vi "GetIntegrationTime.vi"(6 "Delay between send and receive [ms]":i32=100, 8 "error in (no error)":errorcluster, 11 "SCD in":refnum<class "SCD.lvclass">) -> (0 "error out":errorcluster, 2 "integration_time":i32, 3 "SCD out":refnum<class "SCD.lvclass">)   [LabVIEW 2023, in "horiba.lvlib" / "SCD.lvclass"]
doc: "Gets the integration time that was previously set. If no integration time has been explicitly set, the default value is returned.\nThe integration time is returned in seconds."
uses:
  SCD.lvclass
  b6349250-cb33-415b-847a-a7f5d99734f6.vi
  a3575502-22b1-481e-8bb0-96f3cfd6d110.vi
  <vilib>/JDP Science/JSONtext/Variant to JSON Text.vi
  <vilib>/JDP Science/JSONtext/Set Item.vi
  <vilib>/JDP Science/JSONtext/JSON text to Variant.vi
  <vilib>/JDP Science/JSONtext/LVClass Serializer/JSONtext LVClass Serializer.lvclass
  SCD.lvclass/SCD.ctl
  GenericDevice/GenericDevice.lvclass
panel:
  # "Connector Pane"
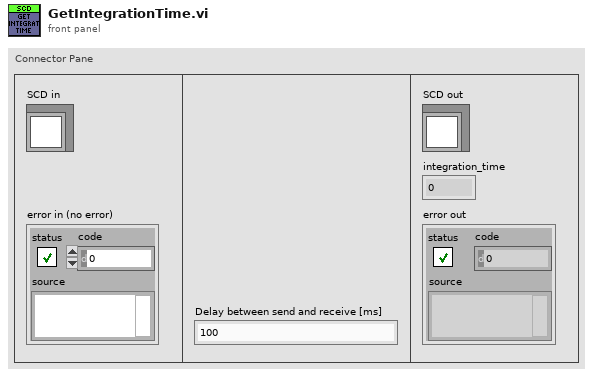
[diagram p1: front panel]
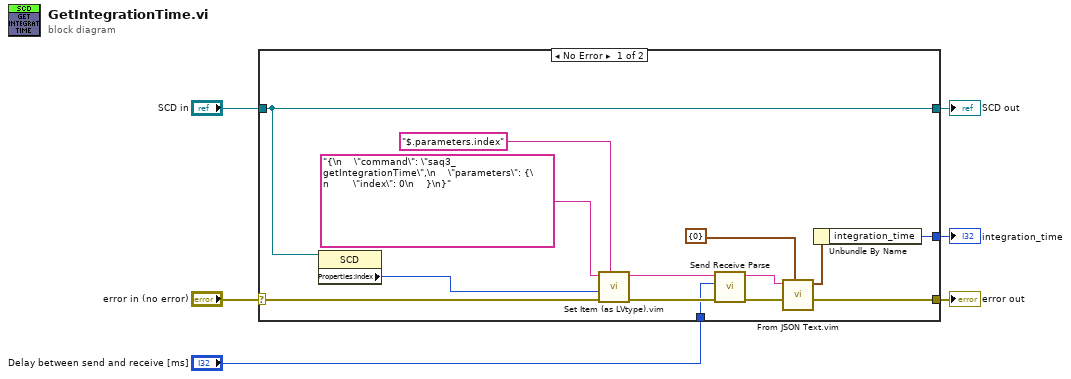
[diagram p0: block diagram]
diagram:
  n1 = case shown="No Error" "error in (no error)" {
    selector: "error in (no error)" -> [w16 w22]
    tunnel: [w15 w22] -> w2
    tunnel: [w18 w21] -> w4
    tunnel: "SCD in" -> [w18 w21]
    tunnel: [w10 _] -> w1
    tunnel: "Delay between send and receive [ms]" -> [w9 _]
    frame No Error {
      n2 = property class="SCD"(reference=w18) -> ("Properties:Index"=w17:i32)  [unwired: 1 in, 2 out]
      n3 = call "Set Item (as LVtype).vim"("$Path or Item Name"="$.parameters.index", "error in (no error)"=w16, "Anything"=w17, "JSON"="{\n    \"command\": \"saq3_getIntegrationTime\",\n    \"parameters\": {\n        \"index\": 0\n    }\n}") -> ("error out"=w13:errorcluster, "<JSON>"=w8:string)  [unwired: 4 in, 1 out]
      n4 = call "Send Receive Parse.vi"("error in"=w13, "Delay between send and receive [ms]"=w9, "<JSON>"=w8) -> ("error out"=w12:errorcluster, "results-JSON string"=w14:string)  [unwired: 6 in, 1 out]
      n5 = call "From JSON Text.vim"("Data Type and Default Value"=cluster{"integration_time":i32} {"integration_time"=0}, "error in (no error)"=w12, "JSON"=w14) -> ("error out"=w15:errorcluster, "Data out"=w11:cluster{"integration_time":i32})  [unwired: 7 in]
      n6 = Unbundle By Name(w11) -> ("integration_time"=w10:i32)
    }
    frame Error {
    }
  }
  "error out" <- w2
  "SCD out" <- w4
  "integration_time" <- w1
